vi "Datasheet Statistics Retrieve Channel Results.vi"(6 "Connection Refnum":T1, 8 "error in (no error)":errorcluster, 9 "Test Parameters":T3, 10 "Grouped Results":cluster{"Result Group":T2[]}[](array[cluster])) -> (0 "error out":errorcluster, 3 "Stat Data":T4)   [LabVIEW 2011]
uses:
  Statistics Data.ctl
  CGI SimpleStat Results.ctl
  Datasheet Analysis Parameters.ctl
  www/cgi-bin/_cgi-lib/TDM_INDEX Record.ctl
  SI.LIB/ODBC/SQL Controls/Connection Refnum.ctl
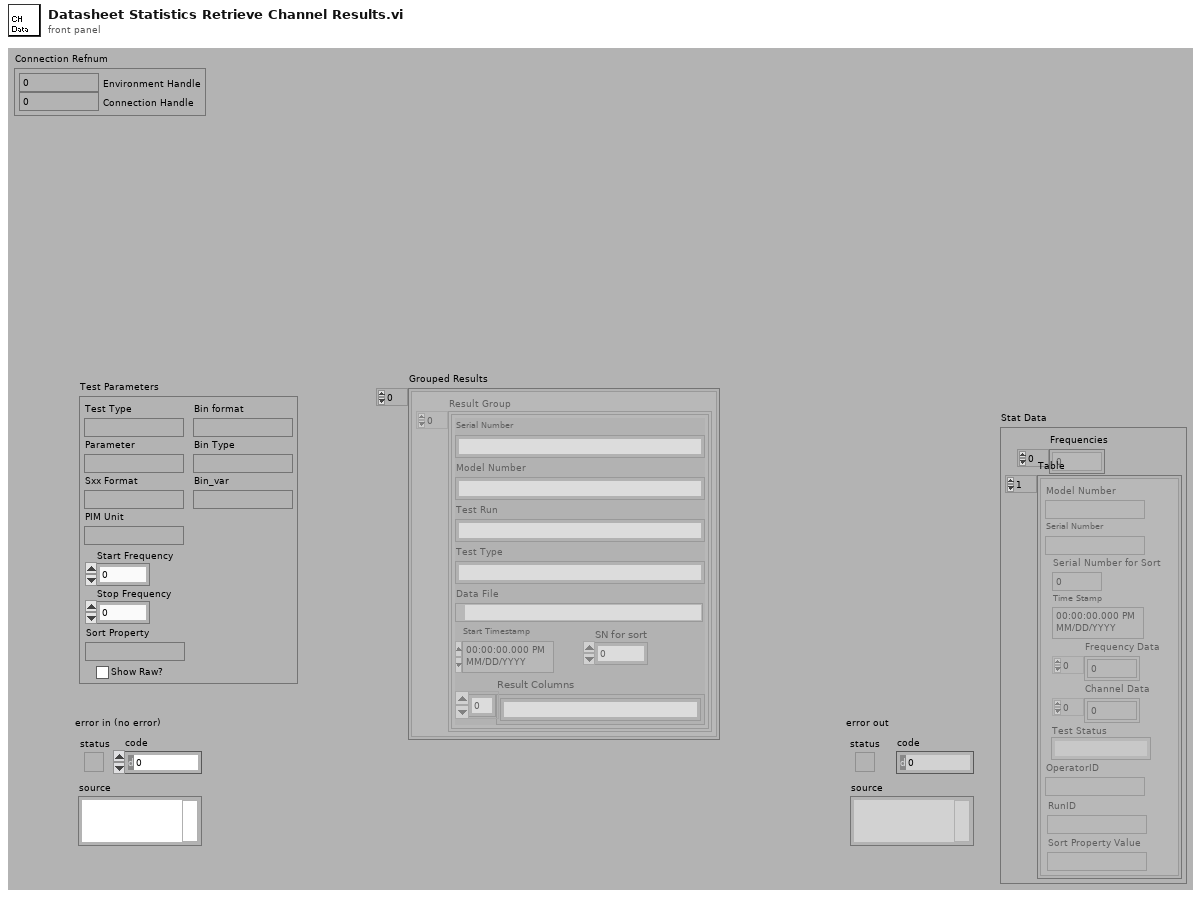
[diagram p1: front panel]
types:
  T1 = typedef "Connection Refnum.ctl" = cluster{"Environment Handle":i32, "Connection Handle":i32}
  T2 = typedef "TDM_INDEX Record.ctl" = cluster{"Model Number":string, "SN for sort":i32, "Test Type":string, "Test Run":string, "Serial Number":string, "Start Timestamp":timestamp, "Data File":path, "Result Columns":string[]}
  T3 = typedef "Datasheet Analysis Parameters.ctl" = cluster{"Test Type":string, "Parameter":string, "Sxx Format":string, "PIM Unit":string, "Start Frequency":dbl, "Stop Frequency":dbl, "Sort Property":string, "Show Raw?":bool, "Bin format":string, "Bin Type":string, "Bin_var":string}
  T4 = typedef "Statistics Data.ctl" = cluster{"Table":T5[], "Frequencies":dbl[]}
  T5 = typedef "CGI SimpleStat Results.ctl" = cluster{"Model Number":string, "Serial Number for Sort":i32, "Serial Number":string, "Time Stamp":timestamp, "Channel Data":dbl[], "Test Status":string, "OperatorID":string, "Frequency Data":dbl[], "RunID":string, "Sort Property Value":string}
  T6 = typedef "Field Record.ctl" = cluster{"ixField":i32, "iSequenceOrder":i32, "sxFieldId":string, "sxSequenceId":string, "sDisplayName":string, "sValue":string, "sUnits":string, "nDataType":T7, "nNextItem":T8, "fSystem":bool, "fSystemValue":bool, "fRequired":bool, "fSetAtTest":bool, "fTestField":bool, "fDeleted":bool, "fIndexed":bool, "fFreeList":bool}
  T7 = typedef "Field DataTypes.ctl" = enum32{"text", "numeric", "list", "timestamp", "boolean"}
  T8 = typedef "Field NextItem.ctl" = enum32{"Reset", "Retain", "Auto-Increment"}
  T9 = typedef "TDMS Model Number.ctl" = cluster{"Model Number":string, "Serial Number Tree Data":T10[]}
  T10 = typedef "TDMS Serial Number.ctl" = cluster{"Serial Number":string, "TDM Files":T11[]}
  T11 = typedef "TDMS File.ctl" = cluster{"File Path":path, "Run Data":T12[], "Serial Number":string, "Model Number":string, "Test Type":string}
  T12 = typedef "TDMS Run.ctl" = cluster{"Channel Data":T13[], "Custom Fields":T6[], "Run ID":string}
  T13 = typedef "TDMS Channel (Sxx).ctl" = cluster{"Channel Name":string, "Waveform":dbl[], "Unit":string, "List value":string}
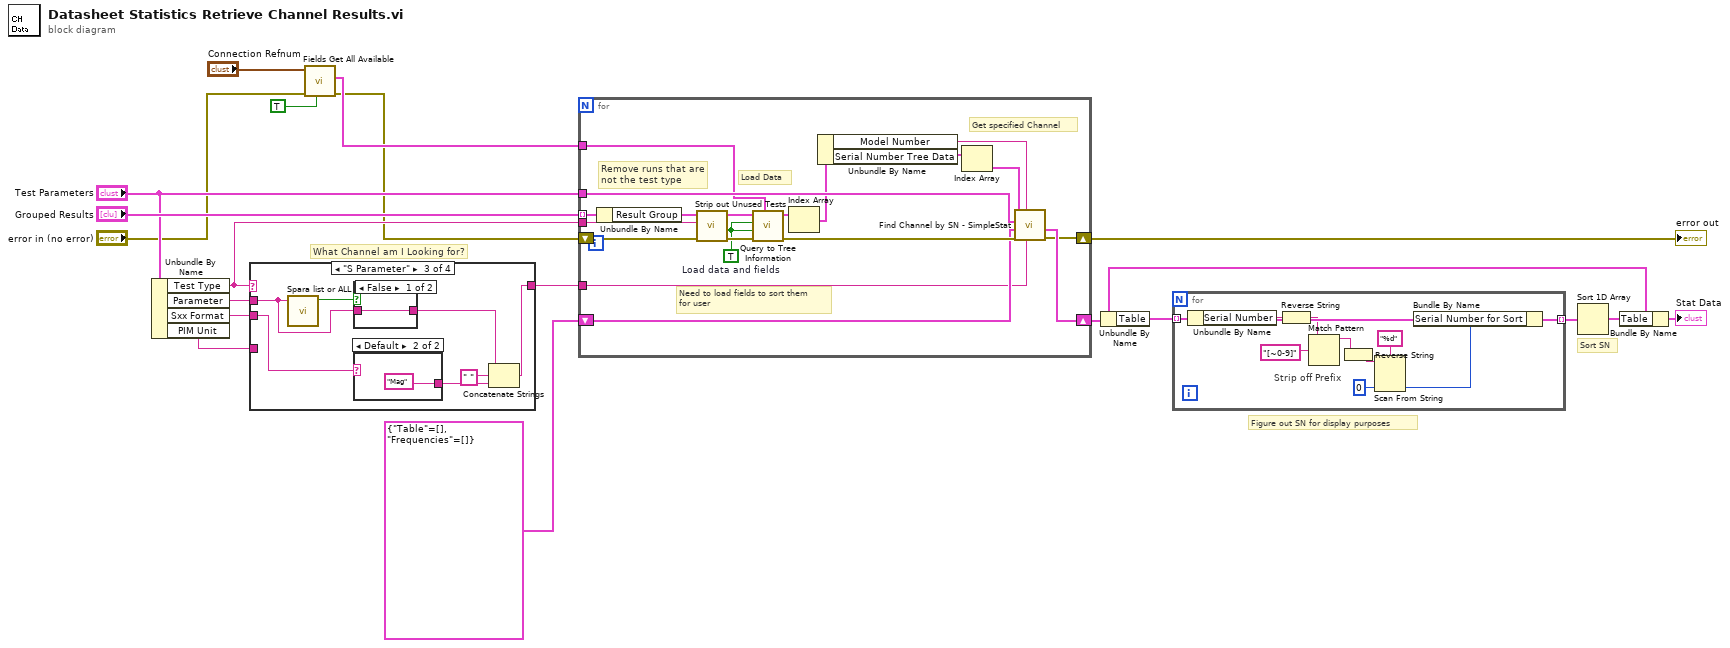
[diagram p0: block diagram]
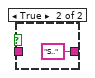
[diagram p4: hidden frame]
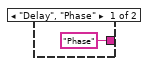
[diagram p5: hidden frame]
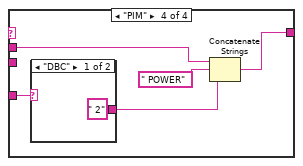
[diagram p6: hidden frame]
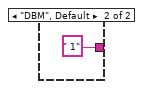
[diagram p7: hidden frame]
diagram:
  # "Sort SN"
  # "Figure out SN for display purposes"
  # "What Channel am I Looking for?"
  n1 = Unbundle By Name("Test Parameters") -> ("Test Type"=w12:string, "Parameter"=w16:string, "Sxx Format"=w15:string, "PIM Unit"=w6:string)
  n2 = case shown="\"S Parameter\"" w12 {
    tunnel: w16 -> [w20 w21 w22 w36]
    tunnel: w15 -> [_ _ w28 _]
    tunnel: [w20 w21 w26 w37] -> w13
    tunnel: w6 -> [_ _ _ w34]
    frame "Prompted Inputs", Default {
      # "For example find Weight in a\nPrompted Inputs tdm File"
    }
    frame "DC Attenuation" {
      # "For example find ATTN in a\nDC Attenuation  tdm File"
    }
    frame "S Parameter" {
      n3 = call "Spara list or ALL.vi"("S## Type"=w22) -> ("S## List or All?"=w23:bool)  [unwired: 10 out]
      n4 = case shown="False" w23 {
        tunnel: [w29 "S.." ("Property Name")] -> w24
        tunnel: w22 -> [w29 _]
        frame False {
        }
        frame True {
        }
      }
      n5 = case shown="Default" w28 {
        tunnel: ["Phase" ("Property Name") "Mag" ("Property Name")] -> w25
        frame "Delay", "Phase" {
        }
        frame Default {
        }
      }
      n6 = Concatenate Strings(w24, " " ("Property Name"), w25) -> (w26:string)
    }
    frame "PIM" {
      n7 = case shown="\"DBC\"" w34 {
        tunnel: [" 2" ("string") " 1" ("string")] -> w33
        frame "DBC" {
        }
        frame "DBM", Default {
        }
      }
      n8 = Concatenate Strings(w36, " POWER" ("string"), w33) -> (w37:string)
    }
  }
  n9 = call "Fields Get All Available.vi"("Combine All? (f)"=TRUE, "error in (no error)"="error in (no error)", "Connection Refnum"="Connection Refnum") -> ("error out"=w2:errorcluster, "System or ALL Combined Fields"=w4:T6[])  [unwired: 3 in, 4 out]
  n10 = for {
    tunnel: "Test Parameters" -> [w49]
    shift-right: [w50] -> w8
    shift-left: T4 {"Table"=[], "Frequencies"=[]} ("Statistics Data") -> [w48]
    shift-right: [w42] -> w18
    shift-left: w2 -> [w56]
    tunnel: "Grouped Results" -> [w57] mode=indexing
    tunnel: w13 -> [w47]
    tunnel: w12 -> [w52]
    tunnel: w4 -> [w40]
    w41 = TRUE  # Load data and fields
    # "Get specified Channel"
    # "Load Data"
    # "Remove runs that are\nnot the test type"
    # "Need to load fields to sort them\nfor user"
    n11 = Unbundle By Name(w57) -> ("Result Group"=w54:T2[])
    n12 = call "Strip out Unused Tests.vi"("error in (no error)"=w56, "Test to remain"=w52, "runs"=w54) -> ("error out"=w55:errorcluster, "runs"=w53:T2[])  [unwired: 7 out]
    n13 = call "Query to Tree Information.vi"("System or ALL Combined Fields"=w40, "error in (no error)"=w55, "Load data? (t)"=w41, "Load Fields? (f)"=w41, "Run Array"=w53) -> ("error out"=w51:errorcluster, "Data Tree"=w58:T9[])  [unwired: 5 out]
    n14 = Index Array(array=w58) -> (element=w46:T9)  [unwired: 1 in]
    n15 = Unbundle By Name(w46) -> ("Model Number"=w43:string, "Serial Number Tree Data"=w45:T10[])
    n16 = Index Array(array=w45) -> (element=w44:T10)  [unwired: 1 in]
    n17 = call "Find Channel by SN - SimpleStat.vi"("Search Channel"=w47, "Model Number"=w43, "error in (no error)"=w51, "Statistics Data"=w48, "Query Parameters"=w49, "Serial Number"=w44) -> ("error out"=w42:errorcluster, "Statistics Data out"=w50:T4)  [unwired: 4 out]
  }
  "error out" <- w18
  n18 = Unbundle By Name(w8) -> ("Table"=w10:T5[])
  n19 = for {
    tunnel: w10 -> [w67] mode=indexing
    tunnel: [w64] -> w11 mode=indexing
    # "Strip off Prefix"
    n20 = Unbundle By Name(w67) -> ("Serial Number"=w62:string)
    n21 = Reverse String(1:w62) -> (0:w61:string)
    n22 = Match Pattern(string=w61, regular expression="[~0-9]" ("format string")) -> (before substring=w59:string)  [unwired: 4 out]
    n23 = Reverse String(1:w59) -> (0:w60:string)
    n24 = Scan From String(format string="%d", input string=w60, default 1=0 ("default value 1")) -> (output 1=w65:i32)  [unwired: 2 in, 3 out]
    n25 = Bundle By Name(cluster=w67, "Serial Number for Sort"=w65) -> (w64:T5)
  }
  n26 = Sort 1D Array(array=w11) -> (sorted array=w9:T5[])
  n27 = Bundle By Name(cluster=w8, "Table"=w9) -> (→"Stat Data":T4)
